vi "DecodeRegisterReply.vi"(2 "error in (no error)":errorcluster, 3 "Response":string="HTTP/1.0 200 OK\r\nServer: BaseHTTP/0.3 Python/2.7.1\r\nDate: Fri, 24 May 2013 07:09:25 GMT\r\nContent-type: text/xml\r\nContent-length: 296\r\n\r\n<?xml version='1.0'?>\n<methodResponse>\n<params>\n<param>\n<value><array><data>\n<value><int>1</int></value>\n<value><string>Unregistered [/labview] as provider of [/robot/head/command_head_nod]</string></value>\n<value><int>1</int></value>\n</data></array></value>\n</param>\n</params>\n</methodResponse>\n") -> (0 "error out":errorcluster, 1 "Reply":T1(array[cluster]))   [LabVIEW 2012]
doc: "Organizes register response into an array of clusters"
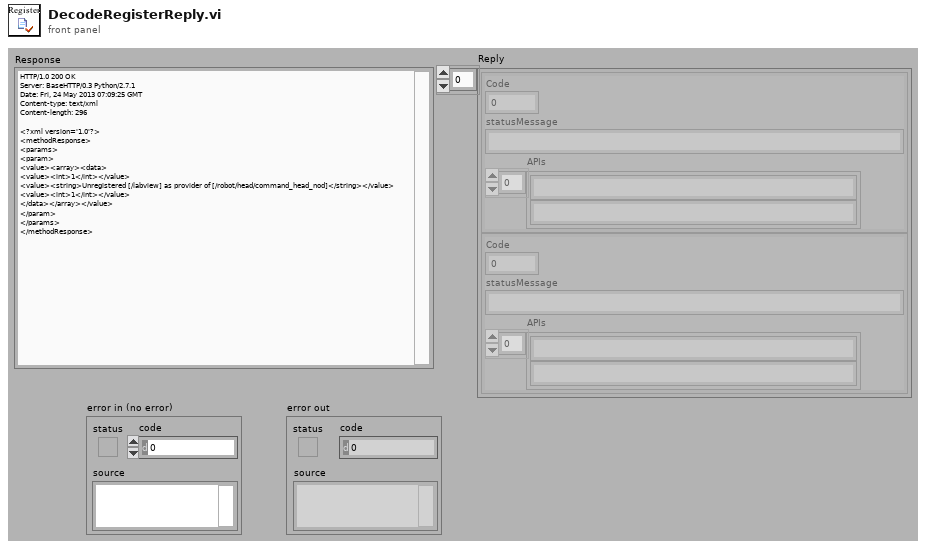
[diagram p1: front panel]
types:
  T1 = cluster{"Code":i8, "statusMessage":string, "APIs":string[]}[]
  T2 = cluster{"Code":i8, "statusMessage":string, "APIs":string[]}
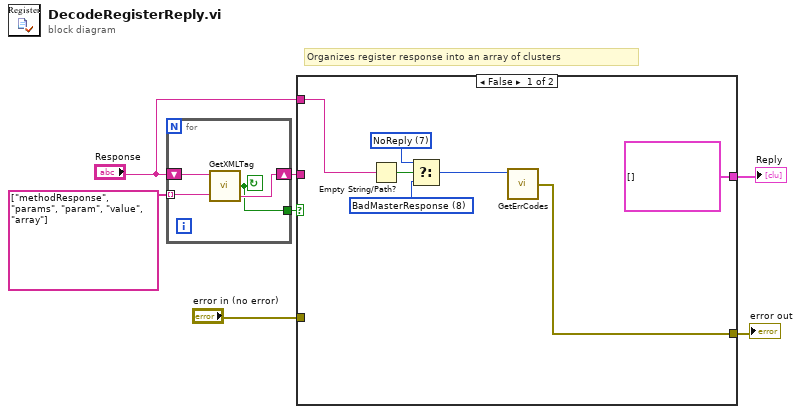
[diagram p0: block diagram]
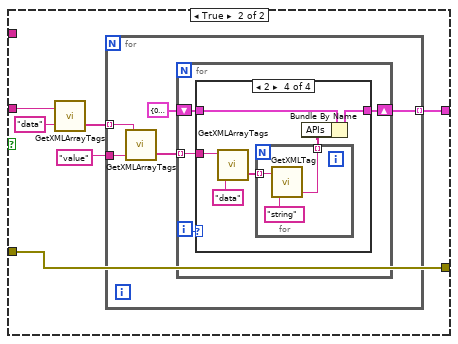
[diagram p2: hidden frame]
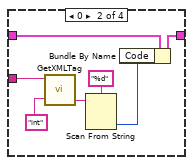
[diagram p4: hidden frame]
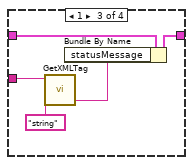
[diagram p5: hidden frame]
diagram:
  # "Organizes register response into an array of clusters"
  n1 = for {
    tunnel: string[] ["methodResponse", "params", "param", "value", "array"] -> [w11] mode=indexing
    shift-right: [w9] -> w6
    shift-left: "Response" -> [w10]
    tunnel: [w8] -> w4
    stop <- w8 continue-if-true
    n2 = call <userlib>:"GetXMLTag.vi"("Tag"=w11, "String"=w10) -> ("Value"=w9:string, "Exists?"=w8:bool)  [unwired: 1 out]
  }
  n3 = case shown="False" w4 {
    tunnel: w6 -> [_ w21]
    tunnel: [T1 [] w20] -> w5
    tunnel: "error in (no error)" -> [_ w19]
    tunnel: [w12 w19] -> w2
    tunnel: "Response" -> [w17 _]
    frame False {
      w15 = u16 8 items=["TopicReadTimeout", "Read=SS", "GetQueueErr", "NoMaster", "Write=PS", "Unparse", "ServiceReply", "NoReply", "BadMasterResponse"] ("Error")
      w14 = u16 7 items=["TopicReadTimeout", "Read=SS", "GetQueueErr", "NoMaster", "Write=PS", "Unparse", "ServiceReply", "NoReply", "BadMasterResponse"] ("Error")
      n4 = Empty String/Path?(string/path=w17) -> (empty?=w16:bool)
      n5 = Select(t=w14, s=w16, f=w15) -> (s? t:f=w13:u16)
      n6 = call <userlib>:"GetErrCodes.vi"("Error"=w13) -> ("Error"=w12:errorcluster)  [unwired: 1 in]
    }
    frame True {
      n7 = call <userlib>:"GetXMLArrayTags.vi"("ArrayTag"="data", "String"=w21) -> ("Array"=w23:string[])  [unwired: 1 out]
      n8 = for {
        tunnel: w23 -> [w29] mode=indexing
        tunnel: "value" -> [w28]
        tunnel: [w25] -> w20 mode=indexing
        n9 = call <userlib>:"GetXMLArrayTags.vi"("ArrayTag"=w28, "String"=w29) -> ("Array"=w27:string[])  [unwired: 1 out]
        n10 = for {
          tunnel: w27 -> [w33] mode=indexing
          shift-right: [w30] -> w25
          shift-left: T2 {"Code"=0, "statusMessage"="", "APIs"=[]} ("Parameters") -> [w31]
          i -> [w32]
          n11 = case shown="2" w32 {
            tunnel: w33 -> [_ w40 w45 w50]
            tunnel: w31 -> [w34 w37 w44 w52]
            tunnel: [w34 w35 w43 w51] -> w30
            frame Default {
            }
            frame 0 {
              n12 = call <userlib>:"GetXMLTag.vi"("Tag"="int", "String"=w40) -> ("Value"=w39:string)  [unwired: 2 out]
              n13 = Scan From String(format string="%d", input string=w39) -> (output 1=w36:i32)  [unwired: 3 in, 3 out]
              n14 = Bundle By Name(cluster=w37, "Code"=w36) -> (w35:T2)
            }
            frame 1 {
              n15 = call <userlib>:"GetXMLTag.vi"("Tag"="string", "String"=w45) -> ("Value"=w42:string)  [unwired: 2 out]
              n16 = Bundle By Name(cluster=w44, "statusMessage"=w42) -> (w43:T2)
            }
            frame 2 {
              n17 = call <userlib>:"GetXMLArrayTags.vi"("ArrayTag"="data", "String"=w50) -> ("Array"=w48:string[])  [unwired: 1 out]
              n18 = for {
                tunnel: w48 -> [w55] mode=indexing
                tunnel: [w53] -> w47 mode=indexing
                n19 = call <userlib>:"GetXMLTag.vi"("Tag"="string", "String"=w55) -> ("Value"=w53:string)  [unwired: 2 out]
              }
              n20 = Bundle By Name(cluster=w52, "APIs"=w47) -> (w51:T2)
            }
          }
        }
      }
    }
  }
  "Reply" <- w5
  "error out" <- w2
